vi "Constants.vi"() -> ()   [LabVIEW 2020, in "SLSC EDS Shared.lvlib"]
doc: "Use this Global VI to access the GUIDs assigned to the page resources of the Custom Device."
uses:
  SLSC EDS Shared.lvlib
panel:
  in  "Tab Control 2":T1(tab)=enum."Properties"
  in  "GUID Get Properties Page":string="c423fa71-92fc-4ef6-9e82-fd6495265e50"
  in  "GUID Command Channel Page":string="93d09459-1801-4e24-92d6-a04ee2d2a9b6"
  in  "GUID Properties Root Page":string="43ced8ca-9492-4202-95f8-a70989870370"
  in  "GUID Properties Section Page":string="c82b20b8-f784-4ce0-9686-ded74c652b63"
  in  "GUID EnableDisable Page":string="99df89e3-c64e-4741-ba8a-793c0469594b"
  in  "GUID Command Page":string="dc60b1f9-7f97-4bba-9f27-d8e24712ca1c"
  in  "GUID Status  Page":string="5eaf23de-b745-4c98-9863-0727b1949205"
  in  "GUID Outgoing Page":string="7097a868-d9b2-4502-84b7-33834e936fb2"
  in  "GUID Incoming Page":string="09e1750a-3fc8-4cf2-bd30-3bfc743a0cd7"
  in  "GUID Main Page":string="8e00a9a9-cfde-4ea5-9266-6ce3d8c7c691"
  in  "GUID Channel Interface":string="e911d720-b8ca-4764-a3ec-6b52f4a67d5a"
  in  "CHM File Name":string="SLSC EDS.chm"
  in  "Channel Interface Name":string="Channel Interface"
  in  "Module.Name":string="SLSC EDS Custom Device"
  in  "product.Num":u32=1
  in  "vendor.Num":u32=1
  in  "CD Version":string="1.1.0"
  in  "Reservation Access":string="Reservation Access"
  in  "Reservation Group":string="Reservation Group"
  in  "SLSC Mod Update Rate":string="SLSC Mod Update Rate"
  in  "ApplyResetOnUndeployment":string="ApplyResetOnUndeployment"
  in  "ApplyValueOnDeployment":string="ApplyValueOnDeployment"
  in  "productNumber":string="productNumber"
  in  "vendorNumber":string="vendorNumber"
  in  "Channel List":string="Channel List"
  in  "Physical Channels":string="Physical Channels"
  in  "Capabilities":string="Capabilities"
  in  "All Properties Name":string="all properties"
  in  "Properties":string="Properties"
  in  "Documentation":string="Documentation"
  in  "capsVersion":string="capsVersion"
  in  "initialized?":string="initialized"
  in  "Command Channel":string="Commands"
  in  "Status Channel":string="Diagnostics"
  in  "Outgoing Channel":string="Outgoing"
  in  "Incoming Channel":string="Incoming"
  in  "SLSCChannelPath":string="SLSCChannelPath"
  in  "PropertyNames":string="PropertyNames"
  in  "Page Configuration Settings":string="Page Configuration Settings"
  in  "Compiled.Settings":string="Compiled.Settings"
  in  "Slot CD Processor Affinity":string="Slot CD Processor Affinity"
  in  "SLSC Root CD Version":string="SLSC Root CD Version"
  in  "SLSC Plug-in Paths":string="SLSC Plug-in Paths"
  in  "SLSC Plug-in GUIDs":string="SLSC Plug-in GUIDs"
  in  "SLSC Plug-in Names":string="SLSC Plug-in Names"
  in  "ModuleName":string="ModuleName"
  in  "Module Number":string="Slot #"
  in  "Chassis #":string="Chassis #"
  in  "Chassis IP Address":string="Chassis IP Address"
  in  "Device.Error.message":string="<not detected or error>"
  in  "SlotX.Property":string="Slot %d.%s"
  in  "Slot CD Name Format":string="Slot %d (SLSC EDS%s)"
  in  "Property.Property":string="%s.%s"
  in  "Config not match msg":string="Configuration file don't match the module on this slot. Do you want to proceed? "
  in  "Cannot Access SLSC msg":string="Host computer can't access the SLSC chassis. Check if the chassis is on and if the IP address is correct. Do you want to check connection to try again?"
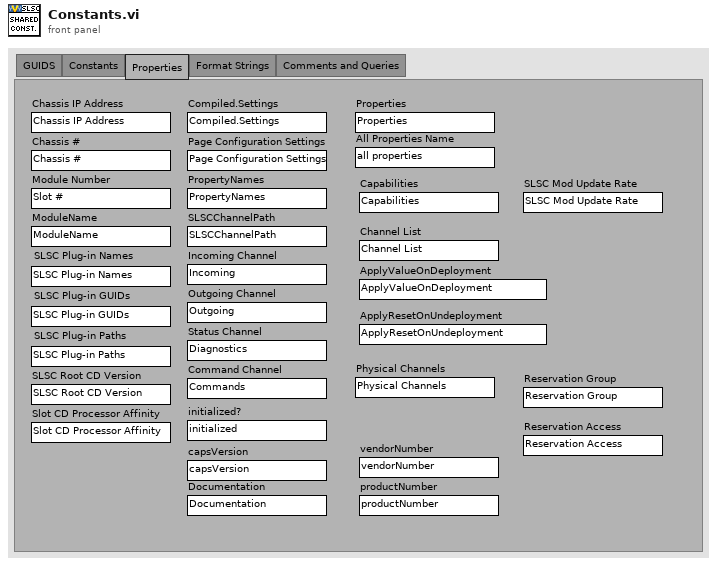
[diagram p1: front panel]
types:
  T1 = enum32{"GUIDS", "Constants", "Properties", "Format Strings", "Comments and Queries"}
diagram:
